vi "Remove Board HW Entry.vi"(10 "boardId":u32, 11 "hw_data in":T1) -> (3 "hw_data out":T1)   [LabVIEW 2020, in "AIM664LV.lvlib"]
uses:
  AIM664LV.lvlib
  _controls/hwEntry_data.ctl
  _controls/hwEntryBoardHandleMap.ctl
  _controls/hwEntryBoardResource.ctl
  _controls/hwEntryPortResource.ctl
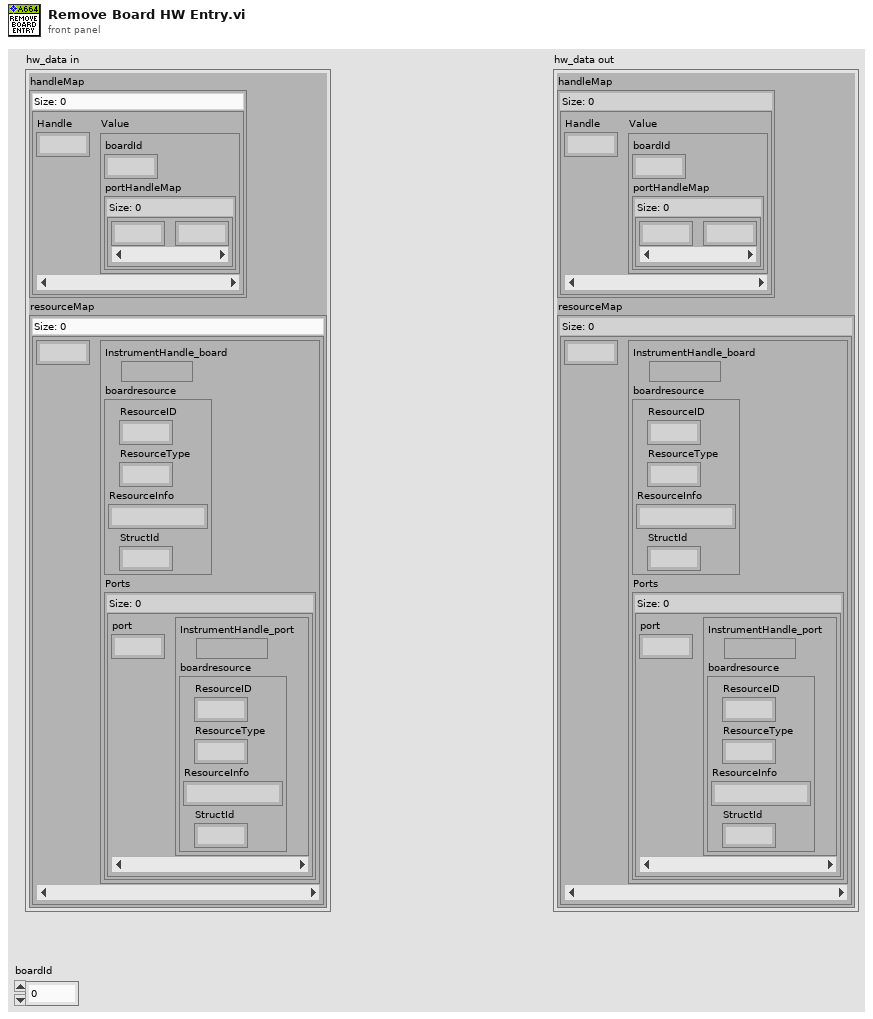
[diagram p1: front panel]
types:
  T1 = typedef "AIM664LV.lvlib/hwEntry_data.ctl" = cluster{"handleMap":map{u32, T2}, "resourceMap":map{u32, T3}}
  T2 = typedef "AIM664LV.lvlib/hwEntryBoardHandleMap.ctl" = cluster{"boardId":u32, "portHandleMap":map{u32, u32}}
  T3 = typedef "AIM664LV.lvlib/hwEntryBoardResource.ctl" = cluster{"InstrumentHandle_board":u32, "boardresource":cluster{"ResourceID":u32, "ResourceType":u32, "ResourceInfo":string, "StructId":u32}, "Ports":map{u32, T4}}
  T4 = typedef "AIM664LV.lvlib/hwEntryPortResource.ctl" = cluster{"InstrumentHandle_port":u32, "boardresource":cluster{"ResourceID":u32, "ResourceType":u32, "ResourceInfo":string, "StructId":u32}}
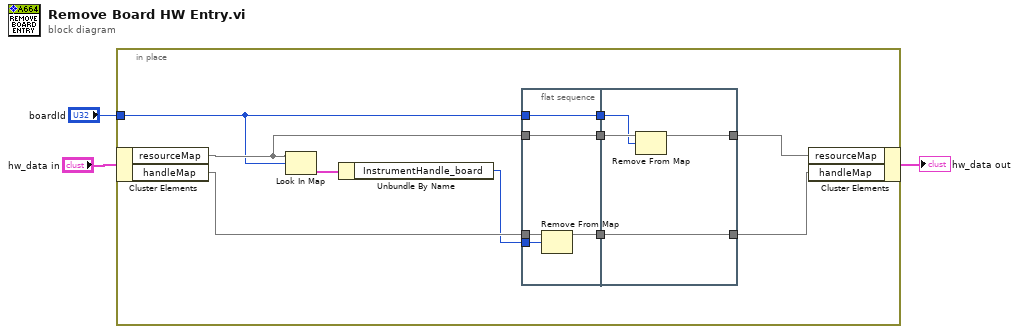
[diagram p0: block diagram]
diagram:
  n1 = in-place {
    in-place-border: "boardId" -> [w5]
    n2 = in-place-cluster #1("hw_data in") -> ("resourceMap"=w7:map{u32, T3}, "handleMap"=w12:map{u32, T2})
    n3 = Look In Map(map=w7, key=w5) -> (value=w13:T3)  [unwired: 1 in, 1 out]
    n4 = Unbundle By Name(w13) -> ("InstrumentHandle_board"=w11:u32)
    n5 = flat-sequence {
      tunnel: w12 -> [w18]
      tunnel: w11 -> [w17]
      tunnel: [w16] -> w9
      tunnel: [w15] -> w8
      tunnel: w7 -> [w15]
      tunnel: [w14] -> w6
      tunnel: w5 -> [w14]
      tunnel: [w22] -> w10
      tunnel: w9 -> [w22]
      tunnel: w8 -> [w21]
      tunnel: w6 -> [w20]
      tunnel: [w19] -> w4
      frame #0 {
        n6 = Remove From Map(10:w17, 11:w18) -> (3:w16:map{u32, T2})  [unwired: 2 out]
      }
      frame #1 {
        n7 = Remove From Map(10:w20, 11:w21) -> (3:w19:map{u32, T3})  [unwired: 2 out]
      }
    }
    n8 = in-place-cluster #1("resourceMap"=w4, "handleMap"=w10) -> (→"hw_data out":T1)
  }
